vi "YOLO11_OBB_OpenVINO.vi"() -> ()   [LabVIEW 2018]
doc: "YOLO11_obb_OpenVINO: This example demonstrates object detection with oriented bounding boxes (OBB) using the YOLO11 algorithm in OpenVINO. The example integrates the object detector model with the OBB extension, enabling the detection of objects along with their orientation in images or videos. By leveraging the YOLO11 architecture's efficiency and accuracy, this example allows for the precise detection of objects, while also providing the ability to estimate their orientation through rotated bounding boxes. The combination of object detection and OBB capabilities allows for more flexible and accurate localization of objects in real-world scenarios where the objects may not be aligned with the axis of the image frame."
uses:
  vi.lib/VIRobotics/ModelZoo/Object_Detection/yolov8_obb_openvino/Initial_yolov8_Obb_OpenVINO.vi
  vi.lib/VIRobotics/opencv_yiku/Cap/Cap.lvclass
  vi.lib/VIRobotics/ModelZoo/Object_Detection/yolov8_obb_openvino/yolov8_obb_openvino.lvclass
  vi.lib/VIRobotics/opencv_yiku/Mat/Mat_8U/Mat_8U.lvclass
panel:
  in  "device_name":string(combo)="CPU"
  in  "config":T1={"confThreshold"=0.3, "nms_threshold"=0.5, "fontScale"=0.5}
  in  "class_names_file":path=path "C:/ProgramData/VIRobotics/ModelZoo/Object_Detection/coco.names"
  in  "model_file":path=path "C:/ProgramData/VIRobotics/ModelZoo/Object_Detection/yolo11_obb/onnx_model/yolo11n-obb.onnx"
  out "picture":picture
  in  "stop":bool
  out "每帧耗时(s)":dbl
  # "Overview: Demonstrates how to use the VIRobotics OpenVINO toolkit to load the the ONNX model of yolo11_obb for real-time object detection.\nRequirements: Windows.\nMake sure your computer has a camera。\nInstructions: \n1.Select the device_name to use.（If your computer has Intel GPU, you can select GPU in the \"type\" control before running the VI to achieve faster inference).\n2.Run the VI.\nIf you want to load the model you trained, follow the following steps:\n1.Select the device_name to use. \n2.Specify the model_file and class_names_file.\n3.Run the VI."
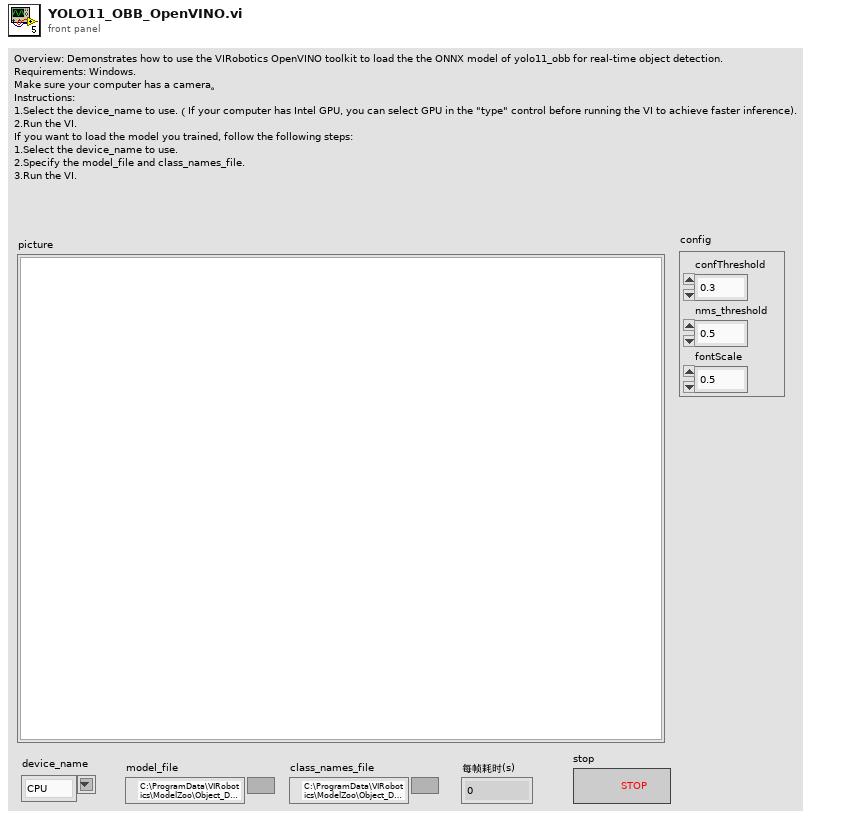
[diagram p1: front panel]
types:
  T1 = cluster{"confThreshold":sgl, "nms_threshold":sgl, "fontScale":dbl}
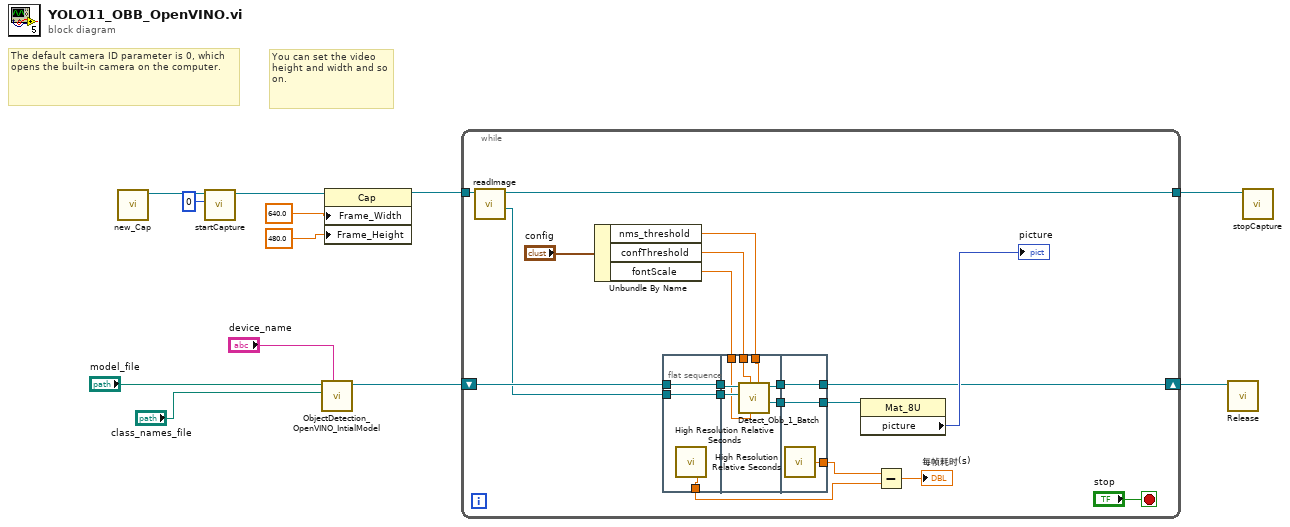
[diagram p0: block diagram]
diagram:
  # "You can set the video height and width and so on."
  # "The default camera ID parameter is 0, which opens the built-in camera on the computer."
  n1 = call "new_Cap.vi"() -> ("Cap out"=w10:refnum<class "Cap.lvclass">)  [unwired: 10 in, 1 out]
  n2 = call "startCapture.vi"("cameraID"=0, "Cap in"=w10) -> ("Cap out"=w7:refnum<class "Cap.lvclass">)  [unwired: 8 in, 1 out]
  n3 = call-poly "ObjectDetection_OpenVINO_IntialModel.vi"("device_name"="device_name", "class_names_path"="class_names_file", "path"="model_file") -> ("yolov8_obb_ov out"=w4:refnum<class "yolov8_obb_openvino.lvclass">)  [unwired: 7 in, 1 out]
  n4 = property class="Cap"(reference=w7, "Frame_Width"=640.0, "Frame_Height"=480.0) -> (reference out=w5:refnum<class "Cap.lvclass">)  [unwired: 1 in, 1 out]
  n5 = while {
    tunnel: w5 -> [w30]
    shift-right: [w26] -> w11
    shift-left: w4 -> [w31]
    tunnel: [w25] -> w12
    stop <- "stop" stop-if-true
    n6 = call "readImage.vi"("Cap in"=w30) -> ("Mat out"=w19:refnum<class "Mat_8U.lvclass">, "Cap out"=w25:refnum<class "Cap.lvclass">)  [unwired: 8 in, 1 out]
    n7 = Unbundle By Name("config") -> ("nms_threshold"=w15:sgl, "confThreshold"=w14:sgl, "fontScale"=w13:dbl)
    n8 = flat-sequence {
      tunnel: w31 -> [w34]
      tunnel: [w34] -> w24
      tunnel: [w33] -> w21
      tunnel: w19 -> [w32]
      tunnel: [w32] -> w18
      tunnel: w24 -> [w40]
      tunnel: [w39] -> w23
      tunnel: w18 -> [w41]
      tunnel: w15 -> [w35]
      tunnel: w14 -> [w36]
      tunnel: w13 -> [w37]
      tunnel: [w38] -> w17
      tunnel: [w43] -> w26
      tunnel: [w44] -> w29
      tunnel: w23 -> [w43]
      tunnel: [w42] -> w22
      tunnel: w17 -> [w44]
      frame #0 {
        n9 = call <vilib>:"High Resolution Relative Seconds.vi"() -> ("relative seconds"=w33:dbl)
      }
      frame #1 {
        n10 = call-dynamic "Detect_Obb_1_Batch.vi"("nms_threshold"=w35, "fontScale"=w37, "confThreshold"=w36, "image"=w41, "yolov8_obb_openvino in"=w40) -> ("image out"=w38:refnum<class "Mat_8U.lvclass">, "yolov8_obb_openvino out"=w39:refnum<class "yolov8_obb_openvino.lvclass">)  [unwired: 3 in, 2 out]
      }
      frame #2 {
        n11 = call <vilib>:"High Resolution Relative Seconds.vi"() -> ("relative seconds"=w42:dbl)
      }
    }
    n12 = property class="Mat_8U"(reference=w29) -> ("picture"=→"picture":picture)  [unwired: 1 in, 2 out]
    n13 = Subtract(x=w22, y=w21) -> (x-y=→"每帧耗时(s)":dbl)
  }
  n14 = call-dynamic "Release.vi"("yolov8_obb_openvino in"=w11) -> ()  [unwired: 9 in, 2 out]
  n15 = call "stopCapture.vi"("Cap in"=w12) -> ()  [unwired: 10 in, 1 out]
